vi "Auth Result.vi"(7 "Session In":refnum<class "Session.lvclass">, 11 "Authentication Outputs":T1) -> (3 "Authentication Result":T1)   [LabVIEW 2020, in "HTTP Server.lvlib" / "Authentication Handler.lvclass"]
uses:
  Authentication Handler.lvclass
  Session/Session.lvclass
  User/User.lvclass
  Authentication Outputs.ctl
  HTTP Server.lvlib
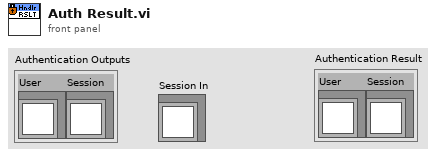
[diagram p1: front panel]
types:
  T1 = typedef "HTTP Server.lvlib/Authentication Outputs.ctl" = cluster{"User":refnum<class "User.lvclass">, "Session":refnum<class "Session.lvclass">}
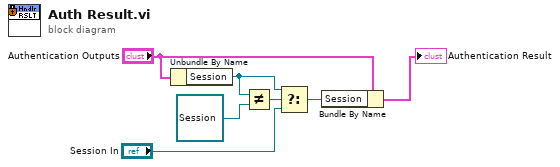
[diagram p0: block diagram]
diagram:
  n1 = Unbundle By Name("Authentication Outputs") -> ("Session"=w4:refnum<class "Session.lvclass">)
  n2 = Not Equal?(x=w4, y=refnum<class "Session.lvclass"> refnum) -> (x != y?=w6:bool)
  n3 = Select(t=w4, s=w6, f="Session In") -> (s? t:f=w2:refnum<class "Session.lvclass">)
  n4 = Bundle By Name(cluster="Authentication Outputs", "Session"=w2) -> (→"Authentication Result":T1)
